vi "CTI_AOTF.vi"(8 "error in":errorcluster, 10 "String":string, 11 "VISA resource name 2":refnum<visa-resource-name>) -> (0 "error out":errorcluster, 2 "read buffer":string)   [LabVIEW 2013]
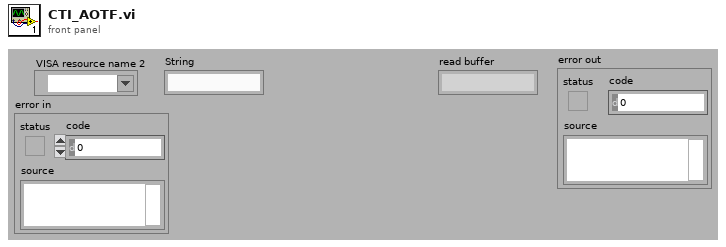
[diagram p1: front panel]
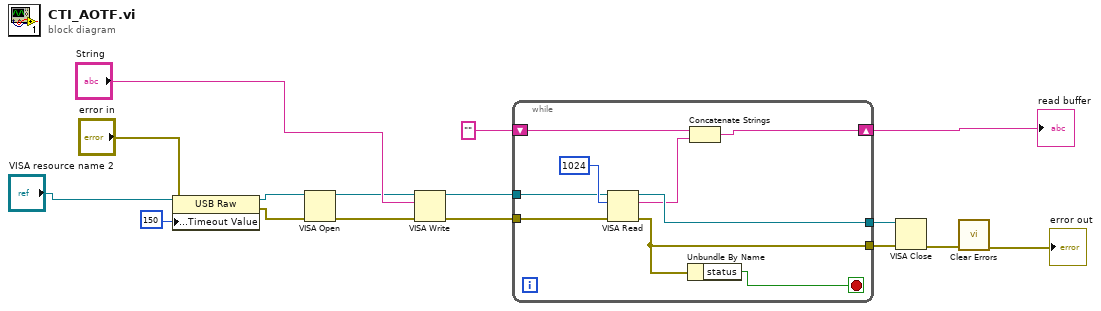
[diagram p0: block diagram]
diagram:
  n1 = property class="USB Raw"(reference="VISA resource name 2", error in="error in", "General Settings:Timeout Value"=u32 150) -> (reference out=w4:refnum<visa-resource-name>, error out=w3:errorcluster)
  n2 = VISA Open(error in (no error)=w3, VISA resource name=w4) -> (VISA resource name=w9:refnum<visa-resource-name>, error out=w8:errorcluster)  [unwired: 3 out]
  n3 = VISA Write(VISA resource name=w9, write buffer="String", error in (no error)=w8) -> (VISA resource name out=w16:refnum<visa-resource-name>, error out=w15:errorcluster)  [unwired: 1 out]
  n4 = while {
    tunnel: w16 -> [w20]
    tunnel: w15 -> [w19]
    shift-right: [w22] -> w13
    shift-left: "" ("read buffer") -> [w25]
    tunnel: [w24] -> w11
    tunnel: [w18] -> w10
    stop <- w17 stop-if-true
    n5 = VISA Read(VISA resource name=w20, byte count=u32 1024, error in (no error)=w19) -> (VISA resource name out=w24:refnum<visa-resource-name>, read buffer=w21:string, error out=w18:errorcluster)  [unwired: 1 out]
    n6 = Unbundle By Name(w18) -> ("status"=w17:bool)
    n7 = Concatenate Strings(w25, w21) -> (w22:string)
  }
  "read buffer" <- w13
  n8 = VISA Close(VISA resource name=w11, error in (no error)=w10) -> (error out=w7:errorcluster)
  n9 = call <vilib>:"Clear Errors.vi"("error in (no error)"=w7) -> ("error out"=→"error out":errorcluster)  [unwired: 6 out]
